vi "Write tcp timeouts.vi"(8 "error in (no error)":errorcluster, 9 "write timeout":i32=10000, 10 "read timeout":i32=10000, 11 "MB_TCP in":refnum<class "Modbus Master CR.lvclass">) -> (0 "error out":errorcluster, 3 "MB_TCP out":refnum<class "Modbus Master CR.lvclass">)   [LabVIEW 2021, in "Modbus Master CR.lvclass"]
uses:
  Modbus Master CR.lvclass
  Modbus Master CR.lvclass/Modbus Master CR.ctl
  Transmission Data Unit/Transmission Data Unit.lvclass
  C:/my_projects/projects/Algorithms/Labview/21/Modbus_v121c/Network Protocol/Network Master/Network Master.lvclass
  C:/my_projects/projects/Algorithms/Labview/21/Modbus_v121c/Network Protocol/Network Protocol.lvclass
  C:/my_projects/projects/Algorithms/Labview/21/Modbus_v121c/Network Protocol/MB/Modbus Master CR.lvclass
  Network Master/Network Master.lvclass
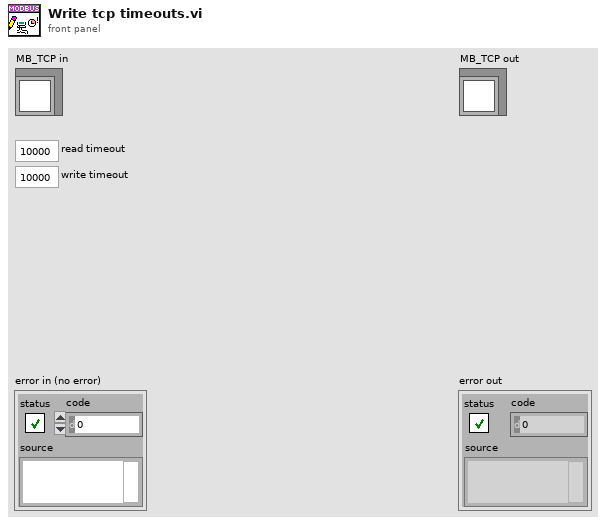
[diagram p1: front panel]
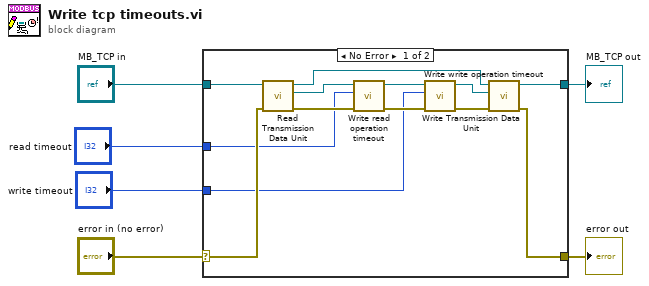
[diagram p0: block diagram]
diagram:
  n1 = case shown="No Error" "error in (no error)" {
    selector: "error in (no error)" -> [w11 w20]
    tunnel: [w7 w20] -> w5
    tunnel: [w8 w21] -> w3
    tunnel: "MB_TCP in" -> [w12 w21]
    tunnel: "read timeout" -> [w10 _]
    tunnel: "write timeout" -> [w9 _]
    frame No Error {
      n2 = call "Read Transmission Data Unit.vi"("error in (no error)"=w11, "Network Master in"=w12) -> ("error out"=w18:errorcluster, "Transmission Data Unit"=w19:refnum<class "Transmission Data Unit.lvclass">, "Network Master out"=w13:refnum<class "Modbus Master CR.lvclass">)  [unwired: 7 in]
      n3 = call "Write read operation timeout.vi"("error in (no error)"=w18, "read operation timeout"=w10, "transmission data unit in"=w19) -> ("error out"=w15:errorcluster, "transmission data unit out"=w16:refnum<class "Transmission Data Unit.lvclass">)  [unwired: 7 in]
      n4 = call "Write write operation timeout.vi"("error in (no error)"=w15, "write operation timeout"=w9, "transmission data unit in"=w16) -> ("error out"=w14:errorcluster, "transmission data unit out"=w17:refnum<class "Transmission Data Unit.lvclass">)  [unwired: 7 in]
      n5 = call "Write Transmission Data Unit.vi"("error in (no error)"=w14, "Transmission Data Unit"=w17, "Network Master in"=w13) -> ("error out"=w7:errorcluster, "Network Master out"=w8:refnum<class "Modbus Master CR.lvclass">)  [unwired: 7 in]
    }
    frame Error {
    }
  }
  "error out" <- w5
  "MB_TCP out" <- w3
